vi "Read gRPC Loop.vi"(8 "error in (no error)":errorcluster, 11 "CIFCorePlugin in":refnum<class "CIFCorePlugin.lvclass">) -> (0 "error out":errorcluster, 2 "gRPC Loop":bool, 3 "CIFCorePlugin out":refnum<class "CIFCorePlugin.lvclass">)   [LabVIEW 2021, in "CIFCorePlugin.lvclass"]
doc: "Indicates if this is being called from inside the gRPC loop. It is used to gate updates in VIs used in both loops such as updating the configuration data."
uses:
  CIFCorePlugin.lvclass
  CIFCorePlugin.lvclass/CIFCorePlugin.ctl
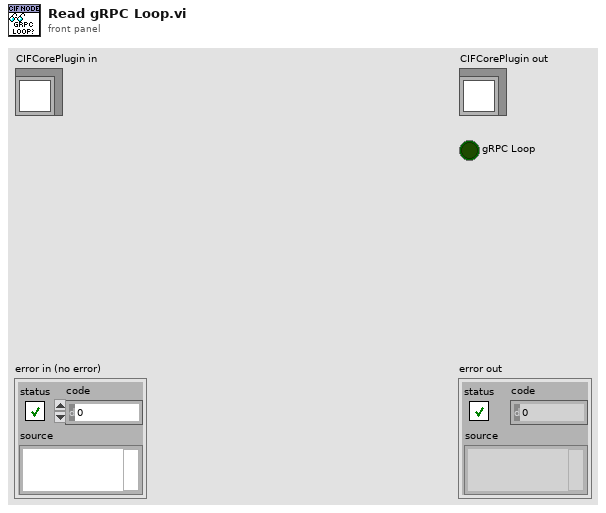
[diagram p1: front panel]
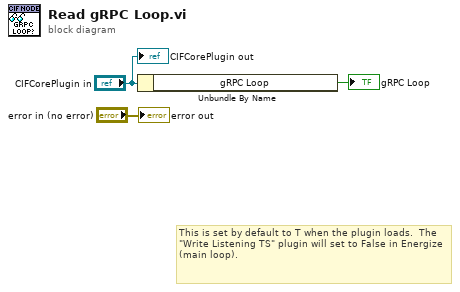
[diagram p0: block diagram]
diagram:
  # "This is set by default to T when the plugin loads.  The \"Write Listening TS\" plugin will set to False in Energize (main loop)."
  n1 = Unbundle By Name("CIFCorePlugin in") -> ("gRPC Loop"=→"gRPC Loop":bool)
  "error out" <- "error in (no error)"
  "CIFCorePlugin out" <- "CIFCorePlugin in"
